vi "Find Distance from Center (SubVI).vi"(5 "Y Center":i16=44, 7 "X Center":i16=5, 10 "Y":u16, 11 "X":u16) -> (3 "Distance from Center":i16)   [LabVIEW 2015]
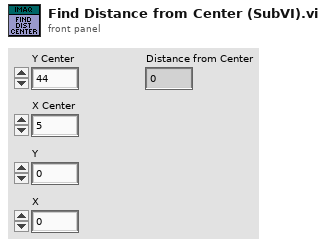
[diagram p1: front panel]
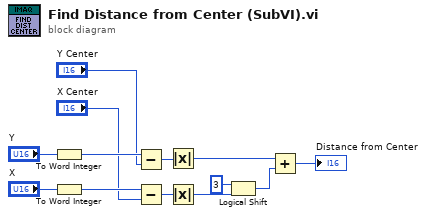
[diagram p0: block diagram]
diagram:
  n1 = To Word Integer(number="Y") -> (16bit integer=w10:i16)
  n2 = To Word Integer(number="X") -> (16bit integer=w9:i16)
  n3 = Subtract(x=w10, y="Y Center") -> (x-y=w8:i16)
  n4 = Subtract(x=w9, y="X Center") -> (x-y=w7:i16)
  n5 = Absolute Value(x=w8) -> (abs(x)=w6:i16)
  n6 = Absolute Value(x=w7) -> (abs(x)=w4:i16)
  n7 = Logical Shift(y=i16 3, x=w4) -> (x << y=w3:i16)
  n8 = Add(x=w6, y=w3) -> (x+y=→"Distance from Center":i16)
